vi "ReadObjectLayout.vi"(7 "properties to ignore":variant, 8 "error in (no error)":errorcluster, 10 "GObj Refnum":refnum<vi>, 11 "Boolean Control Layout in":refnum<class "Boolean Control Layout.lvclass">) -> (0 "error out":errorcluster, 3 "Boolean Control Layout out":refnum<class "Boolean Control Layout.lvclass">)   [LabVIEW 2010, in "NI_SE_Front Panel Layout.lvlib" / "Boolean Control Layout.lvclass"]
doc: "Read layout information from the GObj Refnum."
uses:
  Boolean Control Layout.lvclass
  Control Layout/Control Layout.lvclass
  Boolean Control Layout.lvclass/Boolean Control Layout.ctl
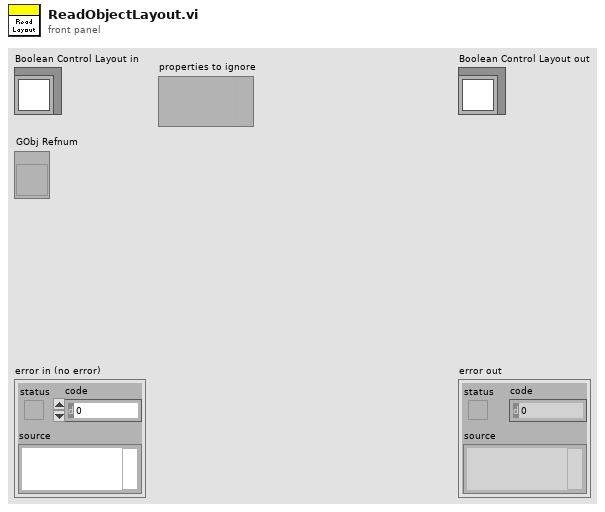
[diagram p1: front panel]
types:
  T1 = typedef "LVFontTypeDef.ctl" = cluster{"Font Name":string, "Size":u16, "Bold":bool, "Italic":bool, "Underline":bool, "Strikeout":bool, "Color":u32}
  T2 = typedef "LVPositionTypeDef.ctl" = cluster{"Left":i32, "Top":i32}
  T3 = typedef "LVBoundsTypeDef.ctl" = cluster{"Width":u32, "Height":u32}
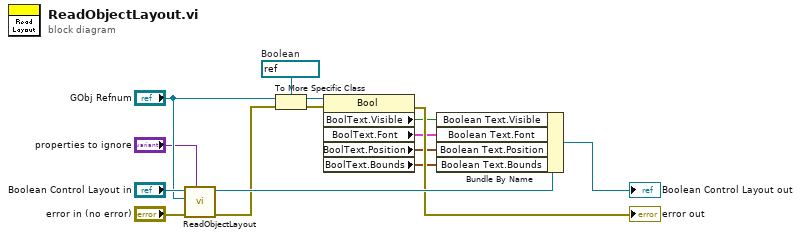
[diagram p0: block diagram]
diagram:
  w7 = refnum<vi> refnum  # Boolean
  n1 = call-parent "ReadObjectLayout.vi"("properties to ignore"="properties to ignore", "error in (no error)"="error in (no error)", "GObj Refnum"="GObj Refnum", "Control Layout in"="Boolean Control Layout in") -> ("error out"=w12:errorcluster, "Control Layout out"=w13:refnum<class "Boolean Control Layout.lvclass">)  [unwired: 6 in]
  n2 = To More Specific Class(target class=w7, reference="GObj Refnum", error in=w12) -> (specific class reference=w6:refnum<vi>, error out=w5:errorcluster)
  n3 = property class="Bool"(reference=w6, error in=w5) -> (error out=→"error out":errorcluster, "BoolText.Visible"=w2:bool, "BoolText.Font"=w3:T1, "BoolText.Position"=w4:T2, "BoolText.Bounds"=w1:T3)  [unwired: 1 out]
  n4 = Bundle By Name(cluster=w13, "Boolean Text.Visible"=w2, "Boolean Text.Font"=w3, "Boolean Text.Position"=w4, "Boolean Text.Bounds"=w1) -> (→"Boolean Control Layout out":refnum<class "Boolean Control Layout.lvclass">)
